vi "Get Supported PIDs.vi"(8 "error in (no error)":errorcluster, 11 "VISA":refnum<visa-resource-name>) -> (0 "error in (no error) 2":errorcluster, 3 "All PIDs":u32[](array[numeric]) format="%x", 4 "transposed array":string[][](array[string]), 6 "Disables":i32[](array[numeric]))   [LabVIEW 2011]
uses:
  PID/PID.lvclass
panel:
  out "Array 2":string[](array[string])
  in  "Multicolumn Listbox":i32(listbox)
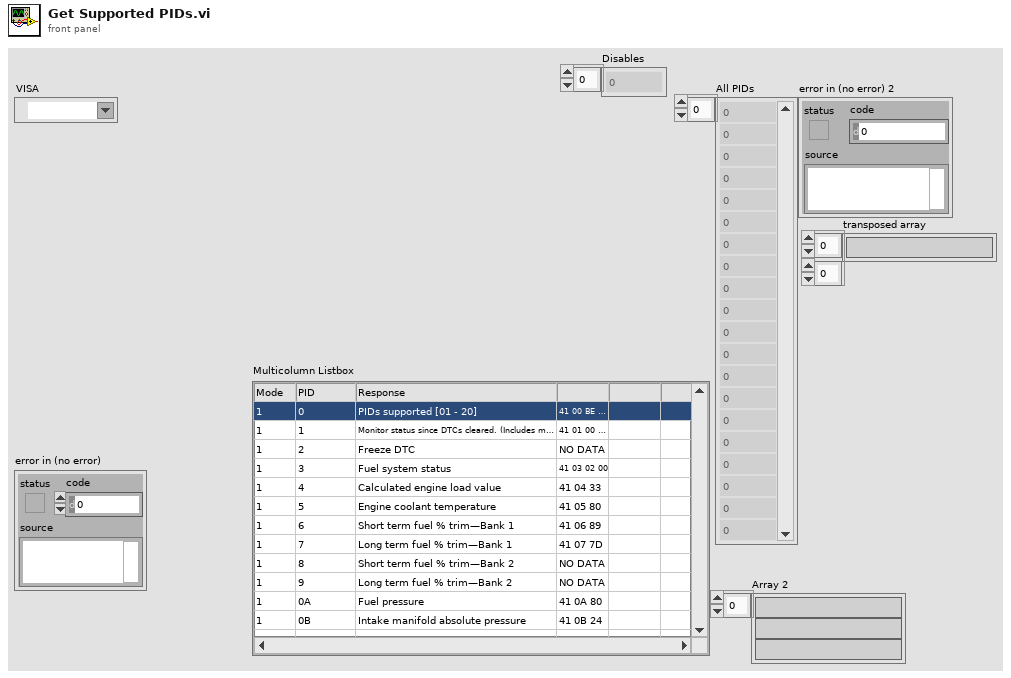
[diagram p1: front panel]
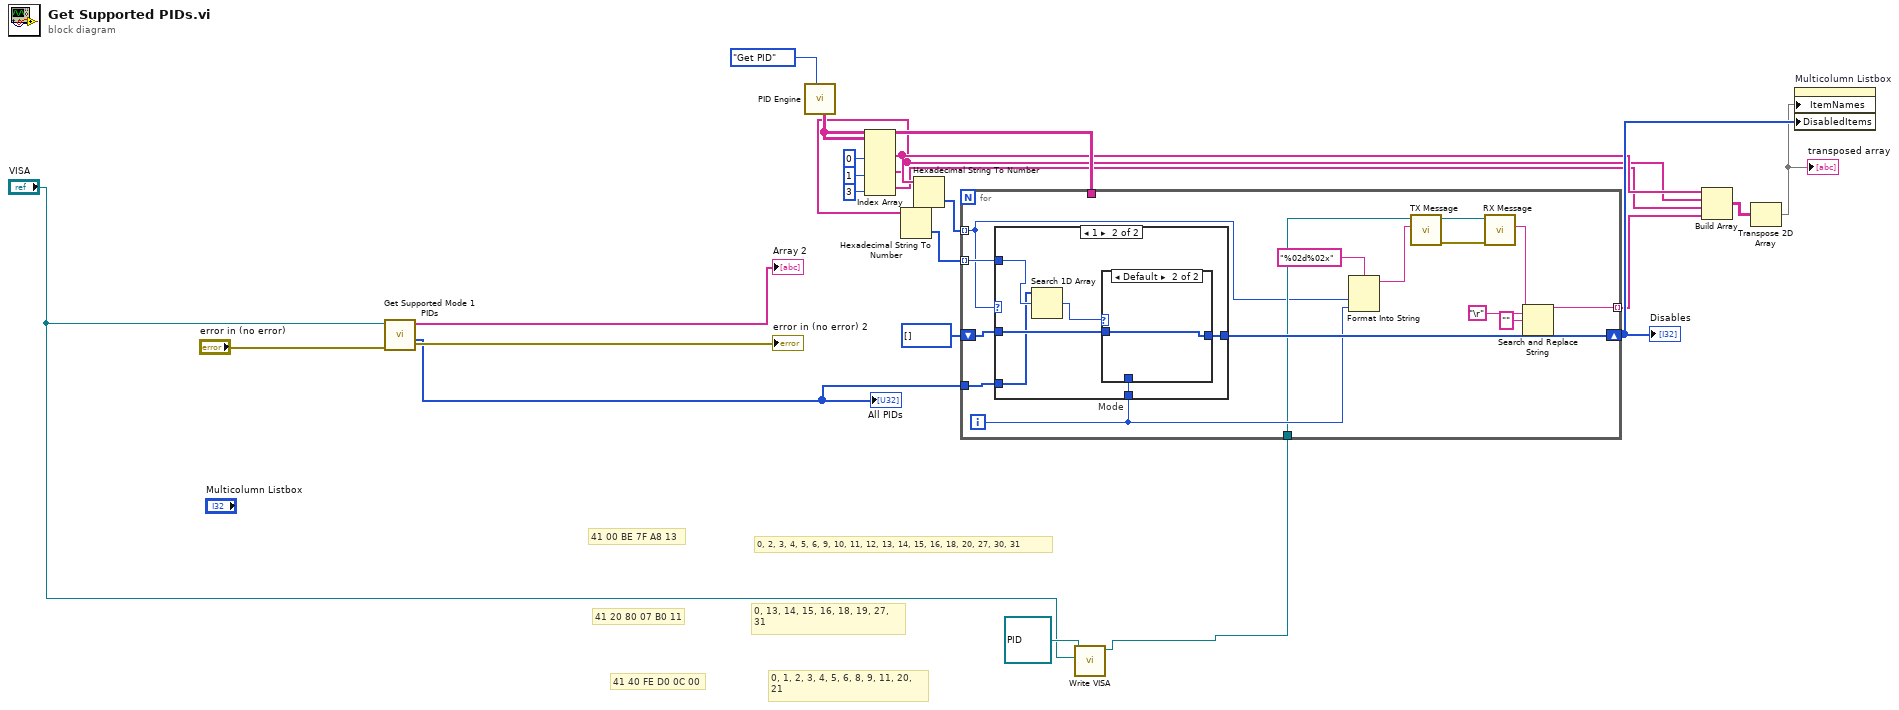
[diagram p0: block diagram]
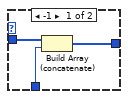
[diagram p3: hidden frame]
diagram:
  # "41 40 FE D0 0C 00"
  # "0, 1, 2, 3, 4, 5, 6, 8, 9, 11, 20, 21"
  # "41 20 80 07 B0 11"
  # "0, 13, 14, 15, 16, 18, 19, 27, 31"
  # "41 00 BE 7F A8 13"
  # "0, 2, 3, 4, 5, 6, 9, 10, 11, 12, 13, 14, 15, 16, 18, 20, 27, 30, 31"
  n1 = call "Get Supported Mode 1 PIDs.vi"("error in (no error)"="error in (no error)", "VISA Refnum in"="VISA") -> ("error out"=→"error in (no error) 2":errorcluster, "Supported PIDs"=w17:u32[], "Array"=→"Array 2":string[])  [unwired: 7 in]
  "All PIDs" <- w17
  n2 = call "PID Engine.vi"("State"=enum16{"Init", "Get PID"}."Get PID") -> ("all rows"=w13:string[][])  [unwired: 7 in, 3 out]
  n3 = Index Array(array=w13, index (col) #1=0 ("disabled index (col)"), index (col) #2=1 ("disabled index (col)"), index (col) #3=3 ("index (col)")) -> (element #1=w4:string[], element #2=w3:string[], element #3=w2:string[])  [unwired: 3 in]
  n4 = Hexadecimal String To Number(string=w3) -> (number=w18:u32[])  [unwired: 2 in, 1 out]
  n5 = Hexadecimal String To Number(string=w4) -> (number=w9:u32[])  [unwired: 2 in, 1 out]
  n6 = call "Write VISA.vi"("VISA"="VISA", "PID in"=refnum<class "PID.lvclass"> refnum ("PID.lvclass")) -> ("PID out"=w8:refnum<class "PID.lvclass">)  [unwired: 8 in, 1 out]
  n7 = for {
    tunnel: w17 -> [w34]
    tunnel: w18 -> [w35] mode=indexing
    tunnel: w13 -> [_]
    shift-right: [w37] -> w11
    shift-left: i32[] [] -> [w36]
    tunnel: w9 -> [w23] mode=indexing
    tunnel: w8 -> [w25]
    tunnel: [w24] -> w7 mode=indexing
    i -> [w26]
    n8 = case "Mode" shown="1" w23 {
      tunnel: w26 -> [_ w43]
      tunnel: [w38 w42] -> w37
      tunnel: w36 -> [w38 w41]
      tunnel: w35 -> [_ w40]
      tunnel: w34 -> [_ w39]
      frame Default {
      }
      frame 1 {
        n9 = Search 1D Array(1D array=w39, element=w40) -> (index of element=w44:i32)  [unwired: 1 in]
        n10 = case shown="Default" w44 {
          tunnel: w43 -> [w47 _]
          tunnel: [w46 w48] -> w42
          tunnel: w41 -> [w45 w48]
          frame -1 {
            n11 = Build Array (concatenate)(w45, w47) -> (w46:i32[])
          }
          frame Default {
          }
        }
      }
    }
    n12 = Format Into String(format string="%02d%02x", w23, w26) -> (resulting string=w28:string)  [unwired: 2 in, 1 out]
    n13 = call-dynamic "TX Message.vi"("variant"=w28, "PID in"=w25) -> ("error out"=w30:errorcluster, "PID out"=w29:refnum<class "PID.lvclass">)  [unwired: 8 in]
    n14 = call-dynamic "RX Message.vi"("error in (no error)"=w30, "PID in"=w29) -> ("String"=w31:string)  [unwired: 7 in, 2 out]
    n15 = Search and Replace String(input string=w31, search string="\r", replace string="" ("replace string (\"\")")) -> (result string=w24:string)  [unwired: 5 in, 3 out]
  }
  "Disables" <- w11
  n16 = Build Array(w4, w3, w2, w7) -> (w1:string[][])
  n17 = Transpose 2D Array(2D array=w1) -> (transposed array=w6:string[][])
  "transposed array" <- w6
  n18 = property on="Multicolumn Listbox" class="MCListbox (strict)"("ItemNames"=w6, "DisabledItems"=w11) -> ()  [unwired: 2 in, 2 out]
